vi "Send MSG.vi"(8 "error in (no error)":errorcluster, 9 "msg value":variant, 10 "msg":string, 11 "UI_ProgressBar in":refnum<class "UI_ProgressDlg.lvclass">) -> (0 "error out":errorcluster, 3 "UI_ProgressBar out":refnum<class "UI_ProgressDlg.lvclass">)   [LabVIEW 2014, in "UI_ProgressDlg.lvlib" / "UI_ProgressDlg.lvclass"]
uses:
  UI_ProgressDlg.lvclass
  UI_ProgressDlg.lvclass/UI_ProgressDlg.ctl
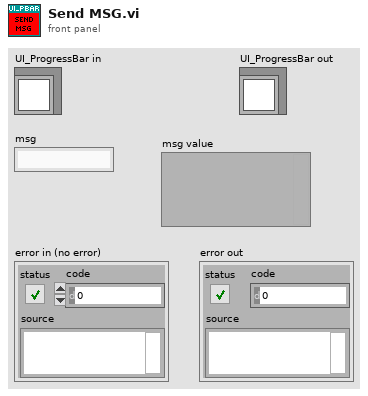
[diagram p1: front panel]
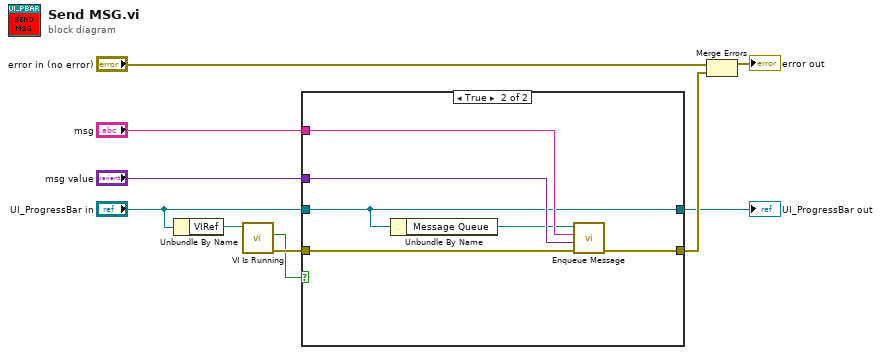
[diagram p0: block diagram]
diagram:
  n1 = Unbundle By Name("UI_ProgressBar in") -> ("VIRef"=w5:refnum<vi>)
  n2 = call "VI Is Running.vi"("VI in"=w5) -> ("error out"=w6:errorcluster, "Running?"=w3:bool)  [unwired: 8 in, 1 out]
  n3 = case shown="True" w3 {
    tunnel: [w12 w16] -> w10
    tunnel: "msg" -> [_ w18]
    tunnel: "msg value" -> [_ w17]
    tunnel: "UI_ProgressBar in" -> [w11 w15]
    tunnel: w6 -> [w12 w14]
    tunnel: [w11 w15] -> w4
    frame False {
    }
    frame True {
      n4 = Unbundle By Name(w15) -> ("Message Queue"=w13:refnum<queue>)
      n5 = call "Enqueue Message.vi"("error in (no error)"=w14, "Message Data"=w17, "Message"=w18, "Message Queue"=w13) -> ("error out"=w16:errorcluster)  [unwired: 6 in, 1 out]
    }
  }
  "UI_ProgressBar out" <- w4
  n6 = Merge Errors("error in (no error)", w10) -> (→"error out":errorcluster)
